vi "RB2 skid steer.vi"() -> ()   [LabVIEW 2012]
uses:
  <vilib>/Utility/inputDevices.llb/closeKeyboard.vi
  <vilib>/Utility/inputDevices.llb/keyboardAcquire.vi
panel:
  out "Speed Balance":i32(knob) scale=-600.0..600.0
  out "IR Volts":dbl
  in  "ESTOP":bool
  in  "Step Size":i32=5
  in  "PC Status":i32=1
  in  "Pan Camera":i32(slide)=1500 scale=500.0..2500.0
  out "Starboard Speed":i32(knob) scale=1150.0..1750.0
  out "Port Speed":i32(knob) scale=1150.0..1750.0
  out "Starboard\nMotor":i32
  out "Port\nMotor":i32
  in  "Rudders":i32(slide)=1500 scale=500.0..2500.0
  out "Right Rubber":i32
  out "Left Rudder":i32
  out "String Received":string
  out "return count":u32
  out "bytes written":u32
  out "Blinky":bool
  in  "String":string="$CS1500P1500R1500L1500P1500H   1\n"
  in  "stop":bool
  in  "VISA resource name":refnum<visa-resource-name>="COM7"
  # "This routine steers the boat using differential thurst as well as the rudders."
  # "USE THE ARROW KEYS TO CHANGE THE MOTOR SPEEDS, UP AND DOWN MOVE TOGETHER, LEFT AND RIGHT ARE DIFFERENTIAL"
  # "Direction of thrust"
  # "DRAG THE SLIDERS TO MOVE THE RUDDER ANGLES AND PAN THE CAMERA."
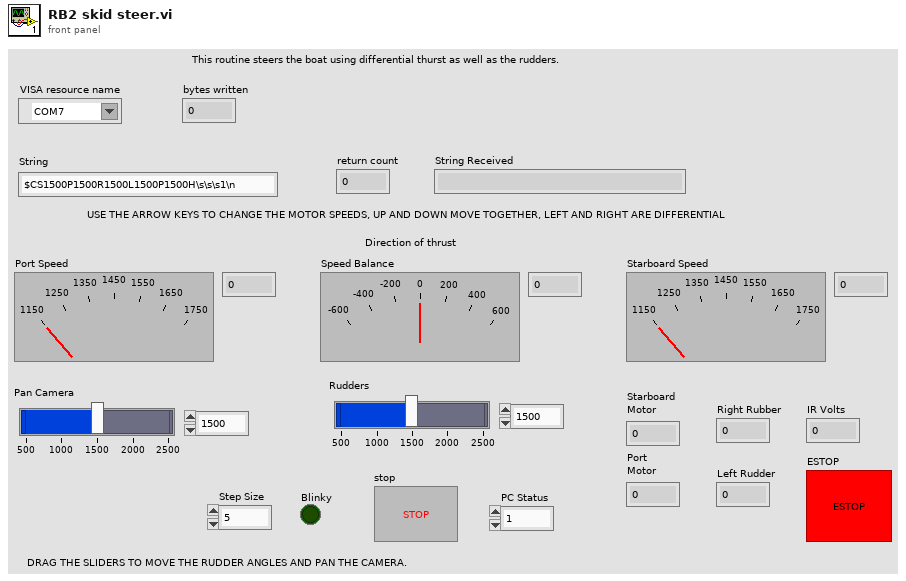
[diagram p1: front panel]
types:
  T1 = enum16{"0", "1", "2", "3", "4", "5", "6", "7", "8", "9", "A", "B", "C", "D", "E", "F", "G", "H", "I", "J", "K", "L", "M", "N", "O", "P", "Q", "R", "S", "T", "U", "V", "W", "X", "Y", "Z", "F1", "F2", "F3", "F4", "F5", "F6", "F7", "F8", "F9", "F10", "F11", "F12", "F13", "F14", "F15", "ADD", "BACK", "BACKSLASH", "CAPITAL", "COMMA", "DECIMAL", "DELETE", "DIVIDE", "DOWN", "END", "EQUALS", "ESCAPE", "GRAVE (`)", "HOME", "INSERT", "LBRACKET", "LCONTROL", "LEFT", "L ALT", "LSHIFT", "LWIN", "MINUS", "MULTIPLY", "NEXT", "NUMLOCK", "NUMPAD_0", "NUMPAD_1", "NUMPAD_2", "NUMPAD_3", "NUMPAD_4", "NUMPAD_5", "NUMPAD_6", "NUMPAD_7", "NUMPAD_8", "NUMPAD_9", "PAUSE", "PERIOD", "PRIOR (PG UP)", "RBRACKET", "RCONTROL", "RETURN", "RIGHT", "R ALT", "RSHIFT", "RWIN", "SCROLL", "SEMICOLON", "SLASH", "SPACE", "SUBTRACT", "TAB", "UP", "ENTER (num pad)", "' (quote)"}[]
  T2 = enum16{"0", "1", "2", "3", "4", "5", "6", "7", "8", "9", "A", "B", "C", "D", "E", "F", "G", "H", "I", "J", "K", "L", "M", "N", "O", "P", "Q", "R", "S", "T", "U", "V", "W", "X", "Y", "Z", "F1", "F2", "F3", "F4", "F5", "F6", "F7", "F8", "F9", "F10", "F11", "F12", "F13", "F14", "F15", "ADD", "BACK", "BACKSLASH", "CAPITAL", "COMMA", "DECIMAL", "DELETE", "DIVIDE", "DOWN", "END", "EQUALS", "ESCAPE", "GRAVE (`)", "HOME", "INSERT", "LBRACKET", "LCONTROL", "LEFT", "L ALT", "LSHIFT", "LWIN", "MINUS", "MULTIPLY", "NEXT", "NUMLOCK", "NUMPAD_0", "NUMPAD_1", "NUMPAD_2", "NUMPAD_3", "NUMPAD_4", "NUMPAD_5", "NUMPAD_6", "NUMPAD_7", "NUMPAD_8", "NUMPAD_9", "PAUSE", "PERIOD", "PRIOR (PG UP)", "RBRACKET", "RCONTROL", "RETURN", "RIGHT", "R ALT", "RSHIFT", "RWIN", "SCROLL", "SEMICOLON", "SLASH", "SPACE", "SUBTRACT", "TAB", "UP", "ENTER (num pad)", "' (quote)"}
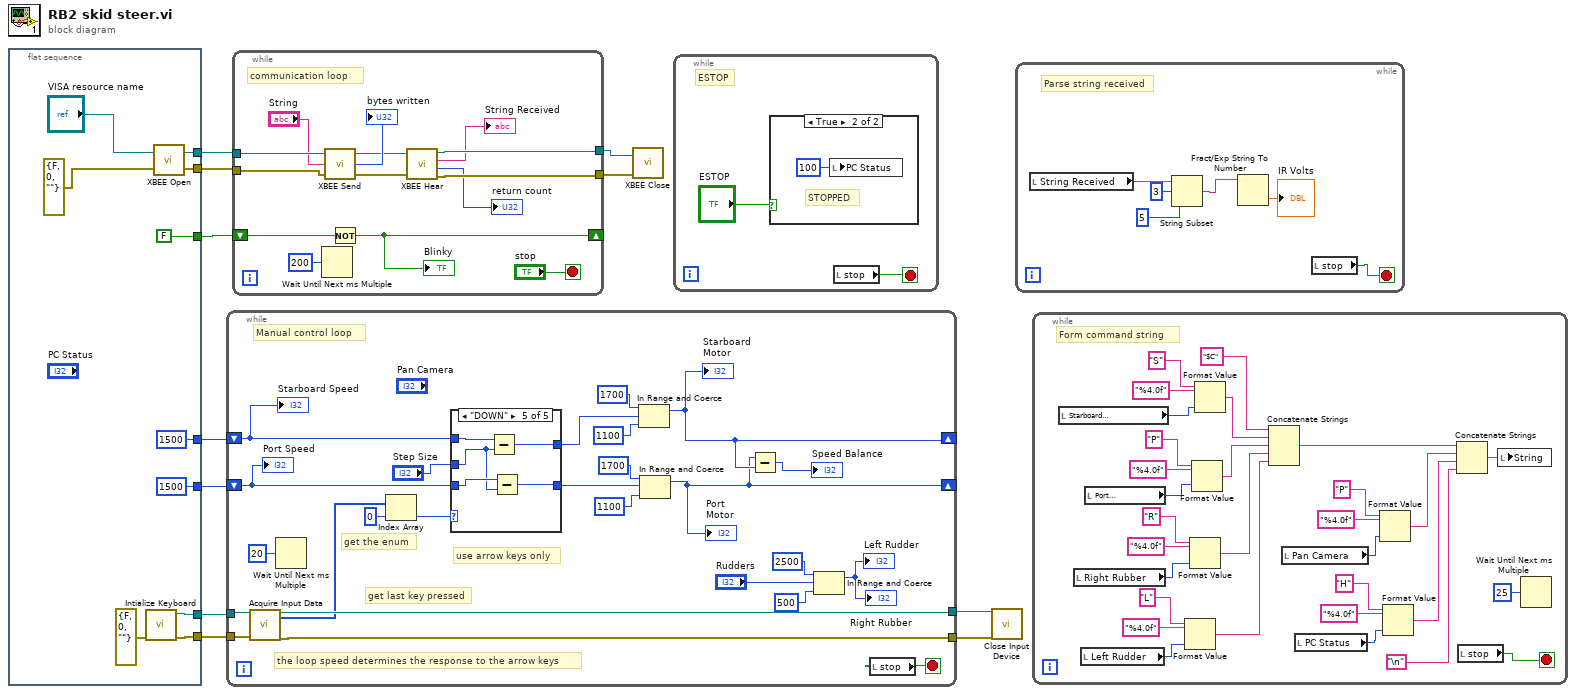
[diagram p0: block diagram]
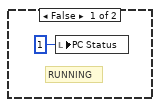
[diagram p2: hidden frame]
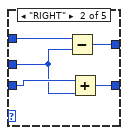
[diagram p4: hidden frame]
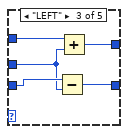
[diagram p5: hidden frame]
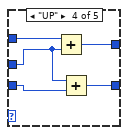
[diagram p6: hidden frame]
diagram:
  n1 = flat-sequence {
    tunnel: [w21] -> w11
    tunnel: [w20] -> w10
    tunnel: [FALSE] -> w7
    tunnel: [w18] -> w6
    tunnel: [w16] -> w5
    tunnel: [1500] -> w2
    tunnel: [1500] -> w1
    frame #0 {
      n2 = call <vilib>:"Intialize Keyboard.vi"("error in (no error)"=errorcluster {"status"=FALSE, "code"=0, "source"=""}) -> ("error out"=w18:errorcluster, "device ID"=w16:refnum<k1>)  [unwired: 9 in]
      n3 = call "XBEE Open.vi"("error in"=errorcluster {"status"=FALSE, "code"=0, "source"=""}, "VISA resource name"="VISA resource name") -> ("error out"=w20:errorcluster, "VISA resource name out"=w21:refnum<visa-resource-name>)
    }
  }
  n4 = while {
    tunnel: w6 -> [w46]
    tunnel: w5 -> [w45]
    tunnel: [w44] -> w4
    tunnel: [w43] -> w3
    shift-right: [w23] -> _
    shift-left: w1 -> [w38]
    shift-right: [w22] -> _
    shift-left: w2 -> [w37]
    stop <- w29 stop-if-true
    # "use arrow keys only"
    # "Manual control loop"
    # "get the enum"
    # "the loop speed determines the response to the arrow keys"
    # "get last key pressed"
    n5 = call-poly <vilib>:"Acquire Input Data.vi"("device ID"=w45, "error in (no error)"=w46) -> ("device ID"=w43:refnum<k1>, "keys pressed"=w42:T1, "error out"=w44:errorcluster)  [unwired: 15 in]
    n6 = Wait Until Next ms Multiple(millisecond multiple=u32 20) -> ()  [unwired: 1 out]
    n7 = Index Array(array=w42, index=0) -> (element=w40:T2)
    n8 = case shown="\"DOWN\"" w40 {
      tunnel: w38 -> [w48 w50 w55 w63 w68]
      tunnel: [w48 w51 w56 w62 w67] -> w36
      tunnel: w37 -> [w47 w53 w57 w60 w66]
      tunnel: [w47 w52 w58 w59 w64] -> w25
      tunnel: "Step Size" -> [_ w49 w54 w61 w65]
      frame "0", Default {
      }
      frame "RIGHT" {
        n9 = Subtract(x=w50, y=w49) -> (x-y=w51:i32)
        n10 = Add(x=w53, y=w49) -> (x+y=w52:i32)
      }
      frame "LEFT" {
        n11 = Subtract(x=w57, y=w54) -> (x-y=w58:i32)
        n12 = Add(x=w55, y=w54) -> (x+y=w56:i32)
      }
      frame "UP" {
        n13 = Add(x=w63, y=w61) -> (x+y=w62:i32)
        n14 = Add(x=w61, y=w60) -> (x+y=w59:i32)
      }
      frame "DOWN" {
        n15 = Subtract(x=w68, y=w65) -> (x-y=w67:i32)
        n16 = Subtract(x=w66, y=w65) -> (x-y=w64:i32)
      }
    }
    n17 = In Range and Coerce(upper limit=1700, x=w36, lower limit=1100) -> (coerced(x)=w23:i32)  [unwired: 1 out]
    "Starboard\nMotor" <- w23
    n18 = In Range and Coerce(upper limit=1700, x=w25, lower limit=1100) -> (coerced(x)=w22:i32)  [unwired: 1 out]
    "Port\nMotor" <- w22
    n19 = Subtract(x=w22, y=w23) -> (x-y=→"Speed Balance":i32)
    n20 = In Range and Coerce(upper limit=2500, x="Rudders", lower limit=500) -> (coerced(x)=→"Right Rubber" →"Left Rudder":i32)  [unwired: 1 out]
    n21 = local read "stop"() -> (w29:bool)
    "Starboard Speed" <- w38
    "Port Speed" <- w37
  }
  n22 = while {
    tunnel: w11 -> [w81]
    tunnel: w10 -> [w80]
    tunnel: [w75] -> w9
    tunnel: [w74] -> w8
    shift-right: [w78] -> _
    shift-left: w7 -> [w79]
    stop <- "stop" stop-if-true
    # "communication loop"
    n23 = Wait Until Next ms Multiple(millisecond multiple=u32 200) -> ()  [unwired: 1 out]
    n24 = call "XBEE Send.vi"("error in (no error)"=w80, "String"="String", "VISA resource name"=w81) -> ("error out"=w71:errorcluster, "return count"=→"bytes written":u32, "VISA resource name out"=w72:refnum<visa-resource-name>)
    n25 = Not(x=w79) -> (.not. x?=w78:bool)
    "Blinky" <- w78
    n26 = call "XBEE Hear.vi"("VISA resource name"=w72, "error in (no error)"=w71) -> ("VISA resource name out"=w75:refnum<visa-resource-name>, "String Received"=→"String Received":string, "return count"=→"return count":u32, "error out"=w74:errorcluster)
  }
  n27 = call "XBEE Close.vi"("error in (no error)"=w8, "VISA resource name"=w9) -> ()
  n28 = while {
    stop <- w84 stop-if-true
    # "ESTOP"
    n29 = case shown="True" "ESTOP" {
      frame False {
        # "RUNNING"
        n30 = local write "PC Status"(1 ("PC Status")) -> ()
      }
      frame True {
        # "STOPPED"
        n31 = local write "PC Status"(100) -> ()
      }
    }
    n32 = local read "stop"() -> (w84:bool)
  }
  n33 = call-poly <vilib>:"Close Input Device.vi"("error in (no error)"=w4, "device ID"=w3) -> ()  [unwired: 8 in, 1 out]
  n34 = while {
    stop <- w89 stop-if-true
    # "Parse string received"
    n35 = local read "String Received"() -> (w92:string)
    n36 = String Subset(string=w92, offset (0)=3, length (rest)=5 ("length (rest)")) -> (substring=w88:string)
    n37 = Fract/Exp String To Number(string=w88) -> (number=→"IR Volts":dbl)  [unwired: 3 in, 1 out]
    n38 = local read "stop"() -> (w89:bool)
  }
  n39 = while {
    stop <- w122 stop-if-true
    # "Form command string"
    n40 = local read "Starboard\nMotor"() -> (w119:i32)
    n41 = local read "Right Rubber"() -> (w110:i32)
    n42 = local read "Left Rudder"() -> (w107:i32)
    n43 = local read "Port\nMotor"() -> (w116:i32)
    n44 = Format Value(string ("")="L", format string="%4.0f", value (0)=w107) -> (output string=w105:string)
    n45 = Format Value(string ("")="R", format string="%4.0f", value (0)=w110) -> (output string=w106:string)
    n46 = Format Value(string ("")="P", format string="%4.0f", value (0)=w116) -> (output string=w113:string)
    n47 = Format Value(string ("")="S", format string="%4.0f", value (0)=w119) -> (output string=w114:string)
    n48 = Concatenate Strings("$C", w114, w113, w106, w105) -> (w97:string)
    n49 = local read "Pan Camera"() -> (w101:i32)
    n50 = local read "PC Status"() -> (w98:i32)
    n51 = Format Value(string ("")="P", format string="%4.0f", value (0)=w101) -> (output string=w96:string)
    n52 = Format Value(string ("")="H", format string="%4.0f", value (0)=w98) -> (output string=w95:string)
    n53 = Concatenate Strings(w97, w96, w95, "\n") -> (w102:string)
    n54 = local read "stop"() -> (w122:bool)
    n55 = local write "String"(w102) -> ()
    n56 = Wait Until Next ms Multiple(millisecond multiple=u32 25) -> ()  [unwired: 1 out]
  }
